vi "RFID TagEvent Example.vi"() -> ()   [LabVIEW 2012, in "Phidget RFID.lvlib"]
uses:
  <instrlib>/Phidgets/Phidget RFID/Phidget RFID.lvlib
  <instrlib>/Phidgets/Phidget RFID/Public/RFIDStart.vi
  <instrlib>/Phidgets/Phidget RFID/Public/RFIDClose.vi
  <instrlib>/Phidgets/Phidget Common/Phidget Common.lvlib
panel:
  out "Protocol":i32(ring) items=["PROTOCOL_EM4100"=1, "PROTOCOL_ISO11785_FDX_B"=2, "PROTOCOL_PHIDGETS"=3]
  out "Tag String":string
  in  "stop":bool
  out "Serial Number Return":i32
  in  "Device Info":T1={"Serial Number"=-1, "Channel"=0, "Port"=0}
  out "error out":errorcluster
  # "Be sure to use this stop button to stop the program.\nIf you use the \"Abort Execution\" button, you will\nneed to use PhidgetResetLibrary.vi or restart Labview \nin order for any Phidgets to work."
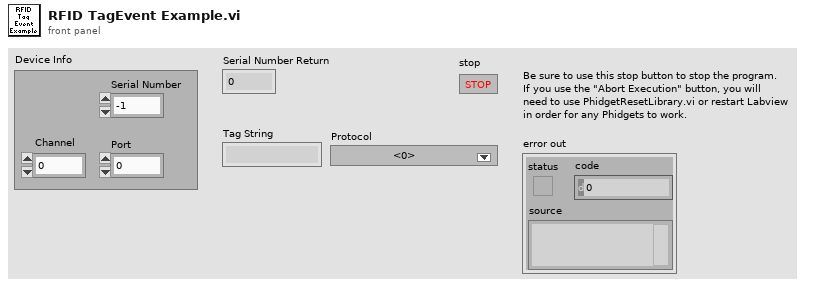
[diagram p1: front panel]
types:
  T1 = cluster{"Serial Number":i32, "Channel":i32, "Port":i32}
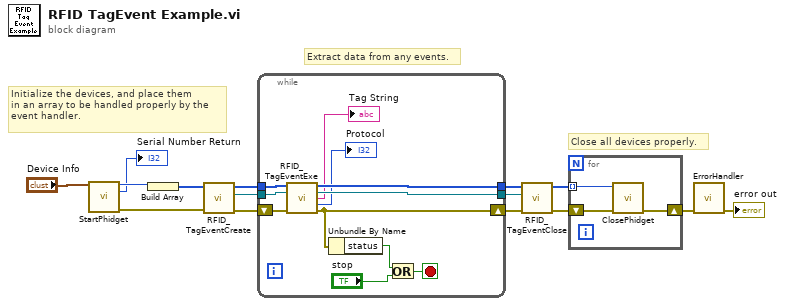
[diagram p0: block diagram]
diagram:
  # "Close all devices properly."
  # "Extract data from any events."
  # "Initialize the devices, and place them\nin an array to be handled properly by the\nevent handler."
  n1 = call-poly <instrlib>:"StartPhidget.vi"("Device Info"="Device Info") -> ("Phidget ID"=w5:u64, "Serial Number Return"=→"Serial Number Return":i32, "error out"=w2:errorcluster)  [unwired: 11 in, 1 out]
  n2 = Build Array(w5) -> (w15:u64[])
  n3 = call <instrlib>:"RFID_TagEventCreate.vi"("error in (no error)"=w2, "Devices In"=w15) -> ("error out"=w8:errorcluster, "Event Registration Refnum Out"=w13:refnum<event-registration>, "Devices Out"=w14:u64[])  [unwired: 7 in]
  n4 = while {
    tunnel: w14 -> [w26]
    tunnel: w13 -> [w22]
    tunnel: [w25] -> w10
    shift-right: [w21] -> w9
    shift-left: w8 -> [w24]
    tunnel: [w23] -> w3
    stop <- w20 stop-if-true
    n5 = call <instrlib>:"RFID_TagEventExe.vi"("Devices In"=w26, "Event Registration Refnum In"=w22, "error in (no error)"=w24) -> ("Devices Out"=w23:u64[], "Event Registration Refnum Out"=w25:refnum<event-registration>, "Tag String"=→"Tag String":string, "Protocol"=→"Protocol":i32, "error out"=w21:errorcluster)  [unwired: 5 in, 3 out]
    n6 = Unbundle By Name(w21) -> ("status"=w18:bool)
    n7 = Or(x=w18, y="stop") -> (x .or. y?=w20:bool)
  }
  n8 = call <instrlib>:"RFID_TagEventClose.vi"("error in (no error)"=w9, "Event Registration Refnum In"=w10, "Devices In"=w3) -> ("error out"=w6:errorcluster, "Devices Out"=w4:u64[])  [unwired: 7 in]
  n9 = for {
    tunnel: w4 -> [w27] mode=indexing
    shift-right: [w29] -> w12
    shift-left: w6 -> [w28]
    n10 = call-poly <instrlib>:"ClosePhidget.vi"("error in"=w28, "Device In"=w27) -> ("error out"=w29:errorcluster)  [unwired: 9 in]
  }
  n11 = call <instrlib>:"ErrorHandler.vi"("error in"=w12) -> ("error out"=→"error out":errorcluster)  [unwired: 9 in, 1 out]
